vi "Write Duty Cycle %.vi"(8 "error in":errorcluster, 10 "Duty Cycle":u8 format="%d %", 11 "IWrite Duty Cycle in":refnum<class "Virtual PWM Generator.lvclass">) -> (0 "error out":errorcluster, 3 "IWrite Duty Cycle out":refnum<class "Virtual PWM Generator.lvclass">)   [LabVIEW 2024, in "Virtual PWM Generator.lvclass"]
uses:
  Virtual PWM Generator.lvclass
  Virtual PWM Generator.lvclass/Virtual PWM Generator.ctl
  Source/Action Point/Action Point.lvclass
  Alarming-Actor/Source/Alarming Actor/Alarming Actor Messages/Update Value Msg/Update Value Msg.lvclass
  D:/git/HAL/Source/Action Point/Action Point.lvclass
  D:/git/HAL/Source/Interfaces/IVirtual Instrument/IVirtual Instrument.lvclass
  D:/git/HAL/Source/Interfaces/IClose/IClose.lvclass
  D:/git/HAL/Source/Interfaces/IHas Configuration/IHas Configuration.lvclass
  D:/git/HAL/Source/Interfaces/IInitialize/IInitialize.lvclass
  D:/git/HAL/Source/Interfaces/IRunnable/IRunnable.lvclass
  D:/git/HAL/HAL-Devices/Source/Virtual Instruments/Virtual PWM Generator/Virtual PWM Generator.lvclass
  D:/git/HAL/Source/Interfaces/IWrite Duty Cycle/IWrite Duty Cycle.lvclass
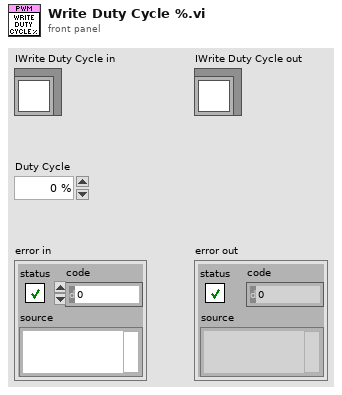
[diagram p1: front panel]
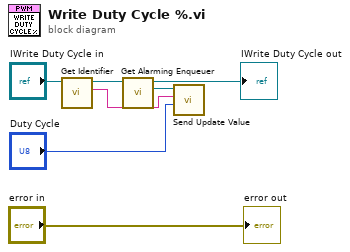
[diagram p0: block diagram]
diagram:
  n1 = call "Get Identifier.vi"("Action Point in"="IWrite Duty Cycle in") -> ("Identifier"=w2:string, "Action Point out"=w3:refnum<class "Virtual PWM Generator.lvclass">)  [unwired: 9 in]
  n2 = call "Get Alarming Enqueuer.vi"("Action Point in"=w3) -> ("Alarming Enqueuer"=w5:refnum<class "Message Enqueuer.lvclass">, "Action Point out"=→"IWrite Duty Cycle out":refnum<class "Virtual PWM Generator.lvclass">)  [unwired: 9 in]
  n3 = call "Send Update Value.vi"("Value"="Duty Cycle", "Identifier"=w2, "Message Enqueuer"=w5) -> ()  [unwired: 7 in, 2 out]
  "error out" <- "error in"
